vi "DataChanged.vi"(9 "Reset data":bool caption="Reset data (F)", 10 "Data":variant) -> (2 "Data changed?":bool)   [LabVIEW 2017, in "GPNumeric.lvlib"]
doc: "**********************************\nTHIS VI HAS BEEN DEPRECATED\n**********************************\n\nUse the IsChanged function from the GPower Comparison v2016.0.0.4 (and newer) library instead.\n\nSteen Schmidt\nGPower\n23/10 2016"
uses:
  GPNumeric.lvlib
panel:
  # "Copyright © 2014\nGPower\nSee enclosed license file for terms and conditions"
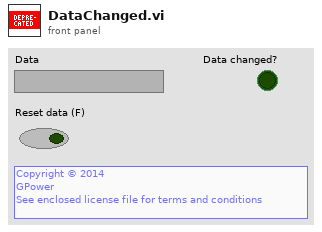
[diagram p1: front panel]
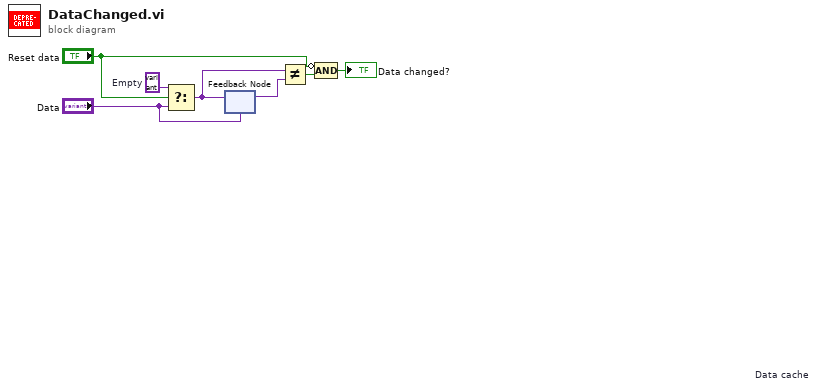
[diagram p0: block diagram]
diagram:
  w6 = variant  # Empty
  n1 = Select(t=w6, s="Reset data", f="Data") -> (s? t:f=w5:variant)
  n2 = feedback-in #1(w5) -> ()
  n3 = feedback #1 "Data cache"("Data") -> (w7:variant)
  n4 = Not Equal?(x=w5, y=w7) -> (x != y?=w3:bool)
  n5 = Compound Arithmetic op=AND(invert "Reset data", w3) -> (→"Data changed?":bool)
